vi "Parse Other Info.vi"(8 "error in (no error)":errorcluster, 10 "SR Cluster in":T1 {"Creation Date" format="%<%x>T"; "Last Updated" format="%<%x>T"}, 11 "remaining string in":string) -> (0 "error out":errorcluster, 2 "SR Cluster out":T1 {"Creation Date" format="%<%x>T"; "Last Updated" format="%<%x>T"}, 3 "result string":string)   [LabVIEW 2018]
uses:
  Type Defs/SR Cluster.ctl
  Type Defs/SR Status.ctl
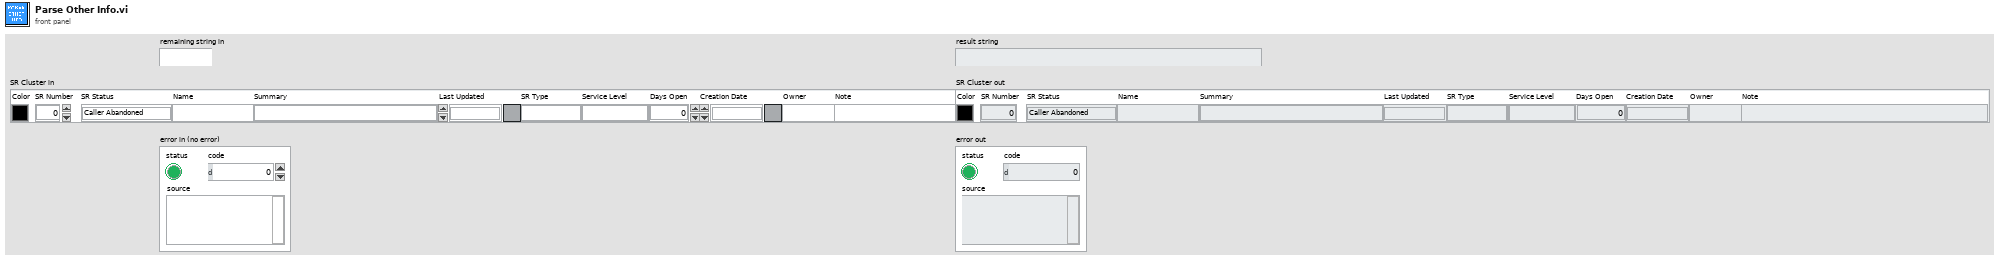
[diagram p1: front panel]
types:
  T1 = typedef "SR Cluster.ctl" = cluster{"Color":u32, "SR Number":i32, "SR Status":T2, "Name":string, "Summary":string, "Last Updated":timestamp, "SR Type":string, "Service Level":string, "Days Open":dbl, "Creation Date":timestamp, "Owner":string, "Note":string}
  T2 = typedef "SR Status.ctl" = enum16{"Caller Abandoned", "Created in Error", "Expired", "Forum Resolved AE", "Forum Resolved Customer", "IN WORK", "IN WORK Collab with AES", "IN WORK Collab with PSE", "IN WORK Collab with SE", "IN WORK Customer Added Note", "IN WORK Escalation", "IN WORK Wait on Customer", "Open", "Potentially Resolved", "Presumed Resolved", "RMA Approved for Return", "RMA Closed", "RMA Closed - DOA", "RMA In Progress", "RMA Open", "RMA Waiting on Customer", "Resolved", "Passed Off"}
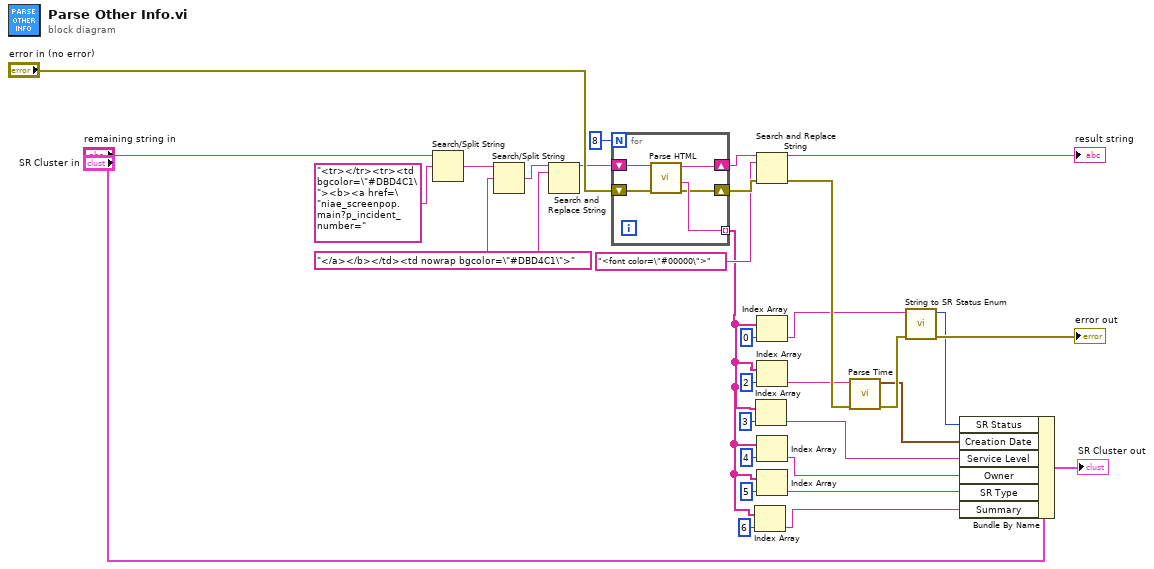
[diagram p0: block diagram]
diagram:
  w8 = "</a></b></td><td nowrap bgcolor=\"#DBD4C1\">" ("search string/char (-)")
  n1 = Search/Split String(string="remaining string in", search string/char (-)="<tr></tr><tr><td bgcolor=\"#DBD4C1\"><b><a href=\"niae_screenpop.main?p_incident_number=") -> (match + rest of string=w11:string)  [unwired: 1 in, 2 out]
  n2 = Search/Split String(string=w11, search string/char (-)=w8) -> (match + rest of string=w9:string)  [unwired: 1 in, 2 out]
  n3 = Search and Replace String(input string=w9, search string=w8) -> (result string=w7:string)  [unwired: 6 in, 3 out]
  n4 = for {
    N: 8 -> [_]
    shift-right: [w36] -> w27
    shift-left: w7 -> [w37]
    tunnel: [w35] -> w3 mode=indexing
    shift-right: [w34] -> w24
    shift-left: "error in (no error)" -> [w33]
    n5 = call "Parse HTML.vi"("error in"=w33, "result string in"=w37) -> ("error out"=w34:errorcluster, "data"=w35:string, "result string out"=w36:string)  [unwired: 7 in]
  }
  n6 = Index Array(array=w3, index=6) -> (element=w1:string)
  n7 = Index Array(array=w3, index=3) -> (element=w19:string)
  n8 = Search and Replace String(input string=w27, search string="<font color=\"#00000\">", error in=w24) -> (result string=→"result string":string, error out=w25:errorcluster)  [unwired: 5 in, 2 out]
  n9 = Index Array(array=w3, index=0) -> (element=w14:string)
  n10 = Index Array(array=w3, index=2) -> (element=w20:string)
  n11 = Index Array(array=w3, index=4) -> (element=w4:string)
  n12 = Index Array(array=w3, index=5) -> (element=w2:string)
  n13 = call "Parse Time.vi"("error in (no error)"=w25, "data"=w20) -> ("error out"=w29:errorcluster, "Time Stamp"=w21:timestamp)  [unwired: 8 in]
  n14 = call "String to SR Status Enum.vi"("error in"=w29, "string in"=w14) -> ("error out"=→"error out":errorcluster, "SR Status"=w15:T2)  [unwired: 8 in]
  n15 = Bundle By Name(cluster="SR Cluster in", "SR Status"=w15, "Creation Date"=w21, "Service Level"=w19, "Owner"=w4, "SR Type"=w2, "Summary"=w1) -> (→"SR Cluster out":T1)
